vi "CHD-simulate-dashboard.vi"() -> ()   [LabVIEW 2019]
uses:
  Differential_Drive_System/CHD_DRIVE_GLOBALS.vi
  Simulation/CHS_SIM_SIM_Globals.vi
  Trajectory Following/CHS_TRAJECTORY_GLOBALS.vi
  Vision_Interface/CHS_Vision_Globals.vi
  <vilib>/Rock Robotics/WPI/ThirdParty/ChoreoLib/ChoreoLib.lvlib
  <vilib>/Rock Robotics/WPI/ThirdParty/JAS_Junk/TrajLib/TypeDef/ROTATION2D.ctl
  <vilib>/Rock Robotics/WPI/ThirdParty/JAS_Junk/TrajLib/Trajectory_Library.lvlib
  <vilib>/Rock Robotics/WPI/ThirdParty/JAS_Junk/TrajLib/TypeDef/CHASSIS_SPEEDS.ctl
  <vilib>/Rock Robotics/WPI/ThirdParty/JAS_Junk/TrajLib/TypeDef/TRANSLATION2D.ctl
  <vilib>/Rock Robotics/WPI/ThirdParty/JAS_Junk/TrajLib/TypeDef/POSE2D.ctl
panel:
  in  "Tab Control":T1(tab)
  out "Battery Voltage":dbl(graph)
  out "Swerve Motor Demands":T2(graph)
  out "Drive Motor Demands":T2(graph)
  out "Swerve Module Devices":T3(array[cluster])
  out "GyroReading_Degreees":dbl format="%15.3f"
  out "Encoder Distances":dbl[](array[numeric]) format="%17.2f"
  out "Encoder Velocities":dbl[](array[numeric]) format="%17.2f"
  out "Motor Demands":dbl[](array[numeric]) format="%17.2f"
  out "Battery Volts":dbl format="%16.2f"
  out "Mod Wheel \nSpeed Dmd":dbl[](array[numeric]) format="%17.3f"
  out "Swerve Drive Motor output":T4(graph)
  out "Drive Wheel Speed M/S":T5(graph)
  out "Swerve Drive Speed Error  M/S":T6(graph)
  out "Closed Loop Control":bool
  out "Orientation Angle Dmd_Rad":dbl format="%17.3f"
  out "Drv Chassis Adj Velocity DmD":T7 {"vOmega" format="%10.3f"; "vY" format="%10.3f"; "vX" format="%10.3f"}
  out "GyroHeading_Radians":dbl format="%17.2f"
  out "Orientation Angle Error_Rad":dbl format="%17.3f"
  out "Orientation Correct CO":dbl format="%17.3f"
  out "Swerve Chassis Speed":T7 {"vOmega" format="%10.3f"; "vY" format="%10.3f"; "vX" format="%10.3f"}
  out "Mod Wheel Out":dbl[](array[numeric]) format="%17.3f"
  out "Drive Wheel Speed M/S":dbl[](array[numeric]) format="%17.3f"
  out "Mod Wheel Speed Err":dbl[](array[numeric]) format="%17.3f"
  out "Mod Wheel \nSpeed Dmd":dbl[](array[numeric]) format="%17.3f"
  out "Closed Loop Control 2":bool
  out "Vision Pose":T8={"TRANSLATION"={"X"=0.0, "Y"=0.0}, "ROTATION"={"VALUE"=0.0, "COS"=1.0, "SIN"=0.0}} {"ROTATION"."SIN" format="%13.4f"; "ROTATION"."COS" format="%13.4f"; "ROTATION"."VALUE" format="%13.4f"; "TRANSLATION"."Y" format="%14.3f"; "TRANSLATION"."X" format="%14.3f"}
  out "Vision\nPose":bool
  out "Trajectory Status":T11(graph)
  out "Trajectory Execution \nClosed Loop":bool
  out "Trajectory Error":T12(graph)
  out "Traj_OnTarget":bool
  out "Traj Heading Dmd Deg":dbl format="%17.2f"
  out "Traj Final Heading Dmd Deg":dbl format="%17.2f"
  out "Traj Sample Time Sec":dbl format="%17.2f"
  out "Traj Rot Vel FF Rad/Sec":dbl format="%17.2f"
  out "Relative Trajectory Pose":T8={"TRANSLATION"={"X"=0.0, "Y"=0.0}, "ROTATION"={"VALUE"=0.0, "COS"=1.0, "SIN"=0.0}} {"ROTATION"."SIN" format="%13.4f"; "ROTATION"."COS" format="%13.4f"; "ROTATION"."VALUE" format="%13.4f"; "TRANSLATION"."Y" format="%14.3f"; "TRANSLATION"."X" format="%14.3f"}
  out "Absolute Odometry \nPose":T8={"TRANSLATION"={"X"=0.0, "Y"=0.0}, "ROTATION"={"VALUE"=0.0, "COS"=1.0, "SIN"=0.0}} {"ROTATION"."SIN" format="%13.4f"; "ROTATION"."COS" format="%13.4f"; "ROTATION"."VALUE" format="%13.4f"; "TRANSLATION"."Y" format="%14.3f"; "TRANSLATION"."X" format="%14.3f"}
  out "Other ABS Odometry\nPose":T8={"TRANSLATION"={"X"=0.0, "Y"=0.0}, "ROTATION"={"VALUE"=0.0, "COS"=1.0, "SIN"=0.0}} {"ROTATION"."SIN" format="%13.4f"; "ROTATION"."COS" format="%13.4f"; "ROTATION"."VALUE" format="%13.4f"; "TRANSLATION"."Y" format="%14.3f"; "TRANSLATION"."X" format="%14.3f"}
  out "Absolue Trajectory":cluster{dbl[], dbl[]}(graph)
  out "Other Trajectory":cluster{dbl[], dbl[]}(graph)
  out "error out":errorcluster
  # "SIMULATION"
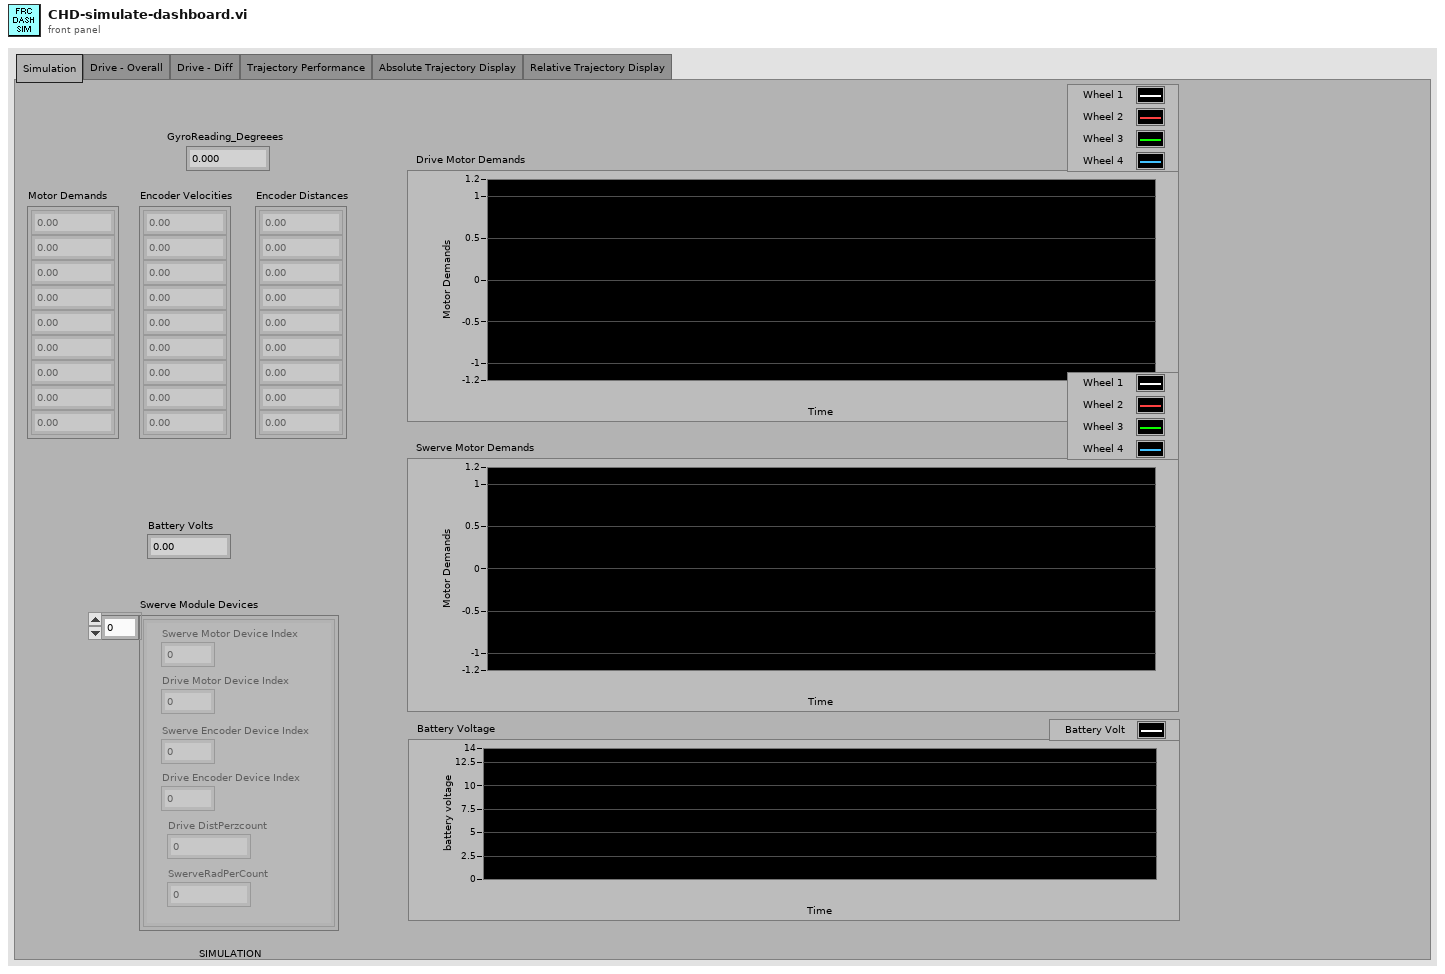
[diagram p1: front panel]
types:
  T1 = enum32{"Simulation", "Drive - Overall", "Drive - Diff", "Trajectory Performance", "Absolute Trajectory Display", "Relative Trajectory Display"}
  T2 = cluster{"Motor Dmd":dbl, "Motor Dmd":dbl, "Motor Dmd":dbl, "Motor Dmd":dbl}
  T3 = cluster{"Swerve Motor Device Index":i32, "Drive Motor Device Index":i32, "Swerve Encoder Device Index":i32, "Drive Encoder Device Index":i32, "Drive DistPerzcount":dbl, "SwerveRadPerCount":dbl}[]
  T4 = cluster{"Mod Wheel Out[0]":dbl, "Mod Wheel Out[1]":dbl, "Mod Wheel Out[2]":dbl, "Mod Wheel Out[3]":dbl}
  T5 = cluster{"LeftSpeed_MperS":dbl, "RightSpeed_MpserS":dbl}
  T6 = cluster{"Mod Wheel Speed Err[0]":dbl, "Mod Wheel Speed Err[1]":dbl, "Mod Wheel Speed Err[2]":dbl, "Mod Wheel Speed Err[3]":dbl}
  T7 = typedef "Trajectory_Library.lvlib/CHASSIS_SPEEDS.ctl" = cluster{"vX":dbl, "vY":dbl, "vOmega":dbl}
  T8 = typedef "Trajectory_Library.lvlib/POSE2D.ctl" = cluster{"TRANSLATION":T9, "ROTATION":T10}
  T9 = typedef "Trajectory_Library.lvlib/TRANSLATION2D.ctl" = cluster{"X":dbl, "Y":dbl}
  T10 = typedef "Trajectory_Library.lvlib/ROTATION2D.ctl" = cluster{"VALUE":dbl, "COS":dbl, "SIN":dbl}
  T11 = cluster{dbl, dbl, dbl, "Traj_Sample_Time_Sec":dbl}
  T12 = cluster{"Traj X Err":dbl, "Traj Y Err":dbl, "Traj Heading Err":dbl}
  T13 = cluster{"Traj X Err_FT":dbl, "Traj Y Err_FT":dbl, "Traj Heading Err_DEG":dbl}
  T14 = typedef "ChoreoLib.lvlib/ChoreoTrajectorySwerve.ctl" = cluster{"name":string, "samples":T15[], "splits":i32[], "events":T16[]}
  T15 = typedef "ChoreoLib.lvlib/ChoreoSwerveSample.ctl" = cluster{"timestamp":dbl, "x":dbl, "y":dbl, "heading":dbl, "velocityX":dbl, "velocityY":dbl, "angularVelocity":dbl, "accelX":dbl, "accelY":dbl, "accelAngular":dbl, "forceX":dbl[], "forceY":dbl[]}
  T16 = typedef "ChoreoLib.lvlib/ChoreoEventMarker.ctl" = cluster{"TimeStamp":dbl, "Name":string}
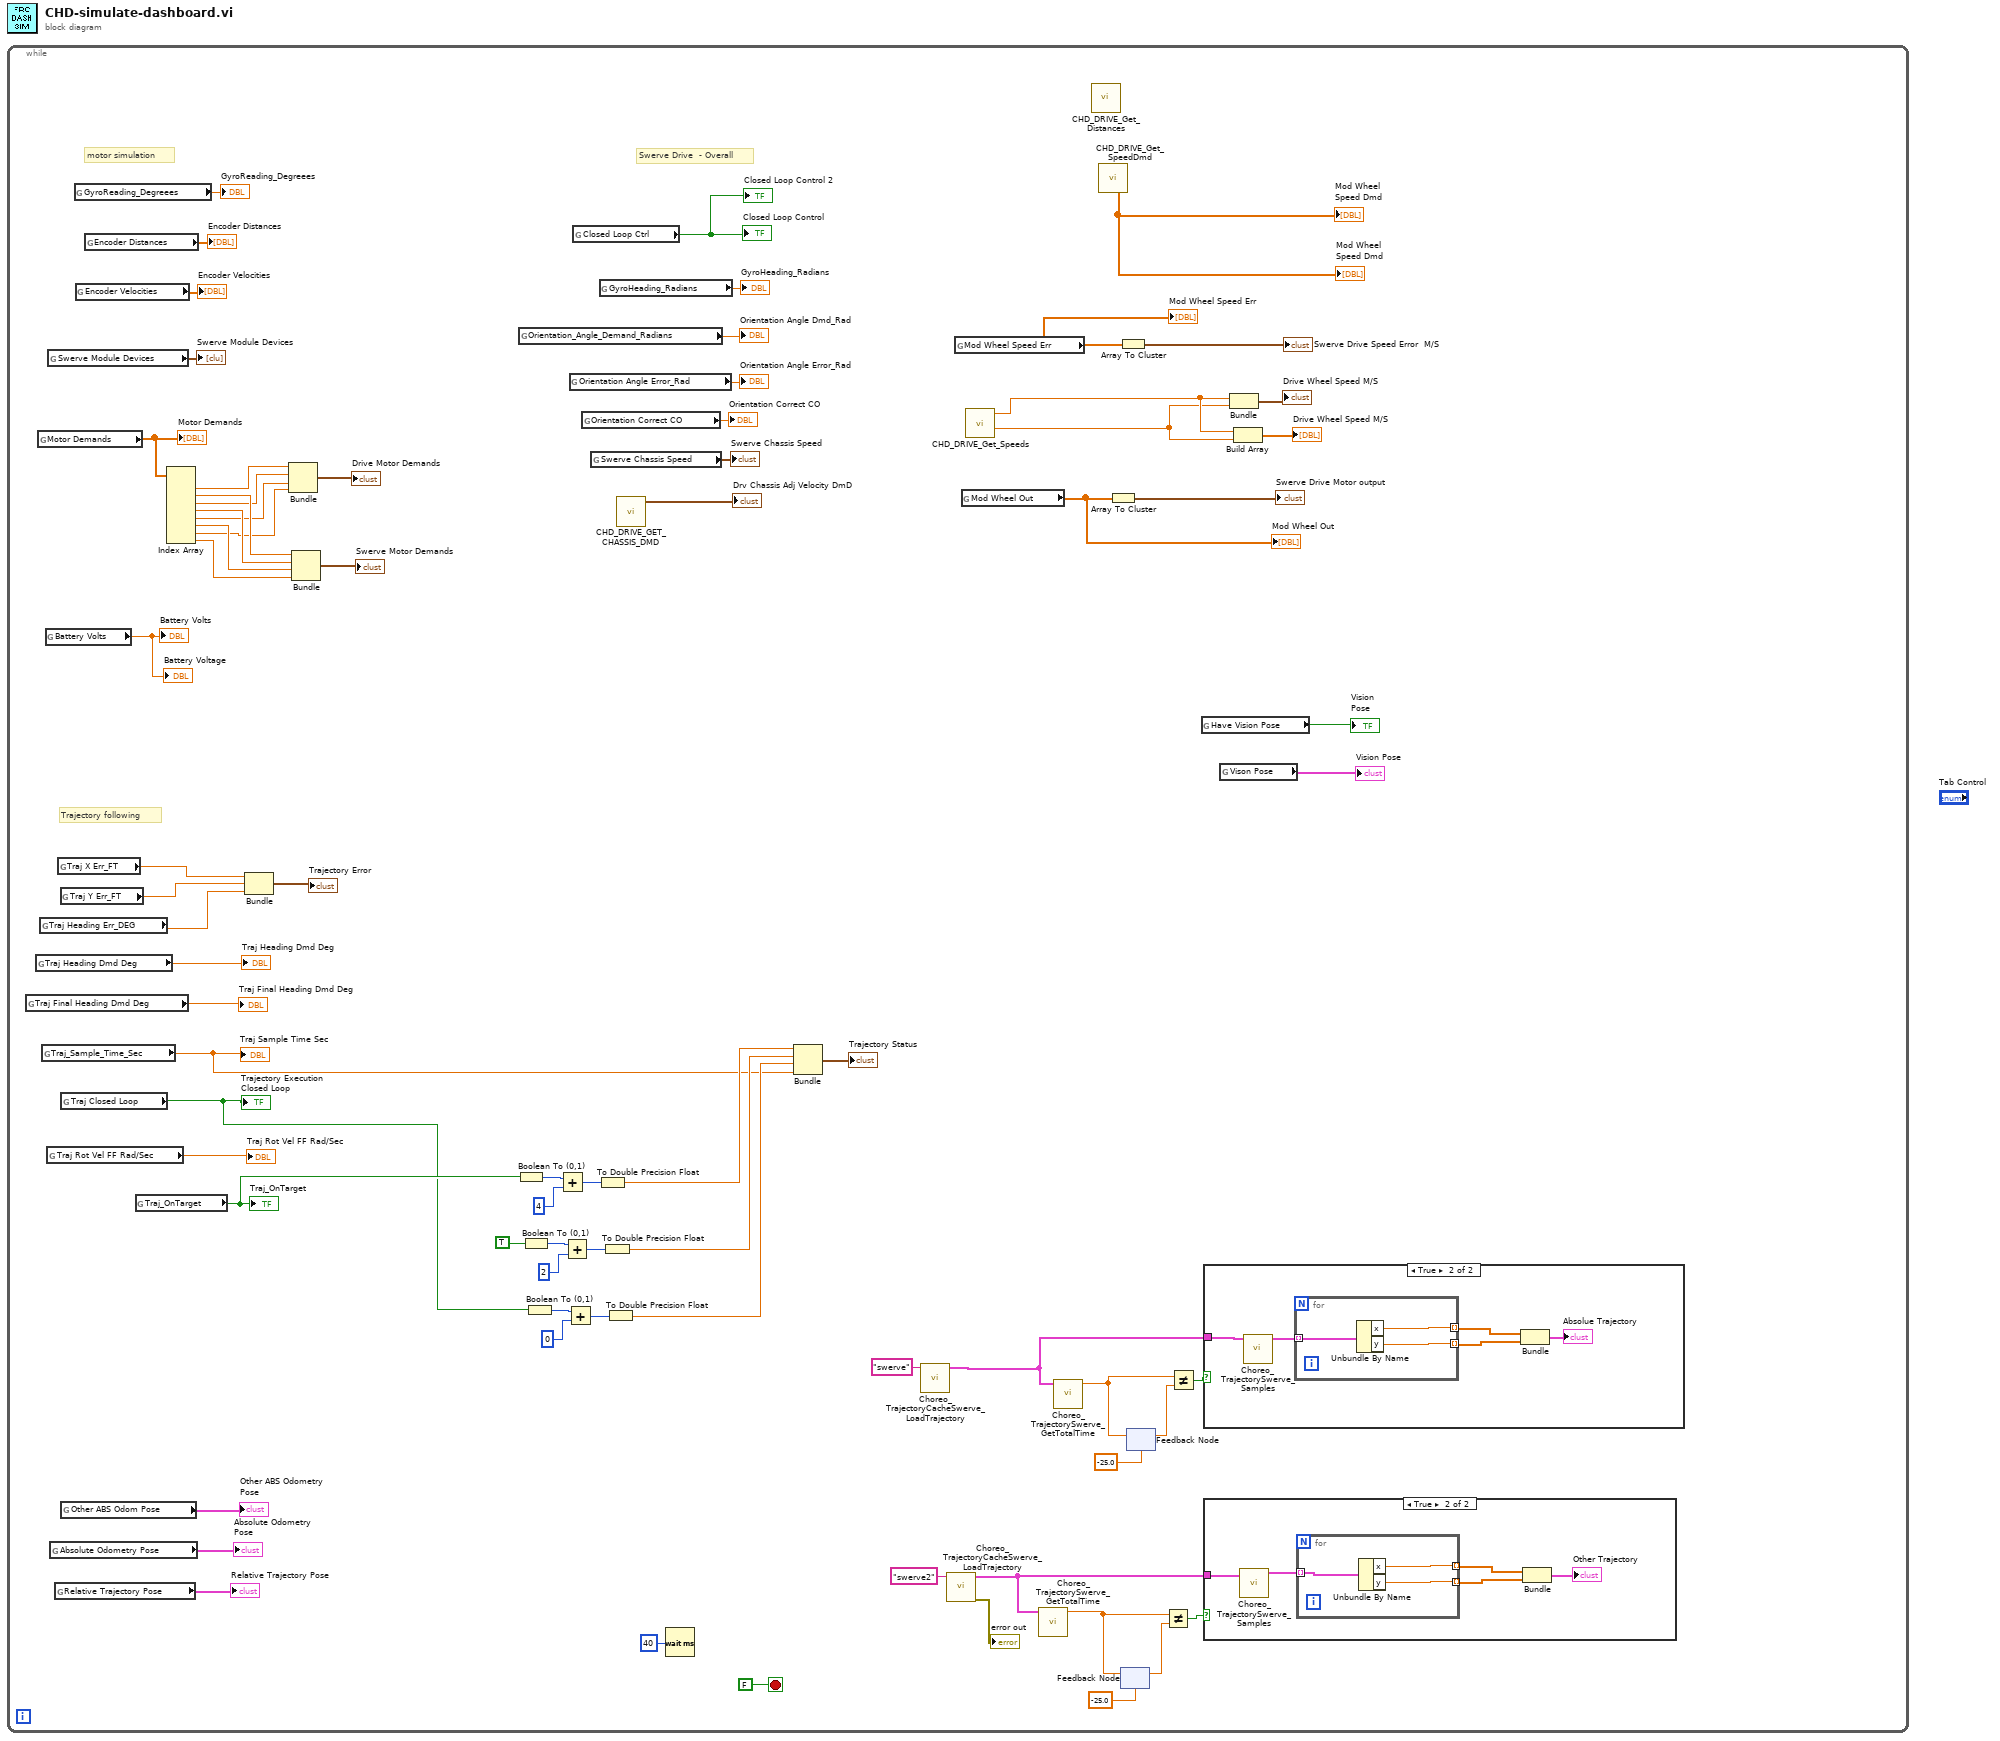
[diagram p0: block diagram]
diagram:
  n1 = while {
    stop <- FALSE stop-if-true
    # "Trajectory following"
    # "motor simulation"
    # "Swerve Drive  - Overall"
    n2 = global read "CHS_TRAJECTORY_GLOBALS.vi" "Traj Final Heading Dmd Deg"() -> (→"Traj Final Heading Dmd Deg":dbl)
    n3 = global read "CHS_TRAJECTORY_GLOBALS.vi" "Traj Heading Dmd Deg"() -> (→"Traj Heading Dmd Deg":dbl)
    n4 = global read "CHS_SIM_SIM_Globals.vi" "Motor Demands"() -> (w63:dbl[])
    "Motor Demands" <- w63
    n5 = global read "CHS_TRAJECTORY_GLOBALS.vi" "Traj Heading Err_DEG"() -> (w50:dbl)
    n6 = global read "CHS_TRAJECTORY_GLOBALS.vi" "Traj_Sample_Time_Sec"() -> (w31:dbl)
    "Traj Sample Time Sec" <- w31
    n7 = global read "CHS_SIM_SIM_Globals.vi" "Battery Volts"() -> (→"Battery Volts" →"Battery Voltage":dbl)
    n8 = global read "CHS_TRAJECTORY_GLOBALS.vi" "Traj Rot Vel FF Rad/Sec"() -> (→"Traj Rot Vel FF Rad/Sec":dbl)
    n9 = global read "CHS_SIM_SIM_Globals.vi" "Swerve Module Devices"() -> (→"Swerve Module Devices":T3)
    n10 = global read "CHS_TRAJECTORY_GLOBALS.vi" "Absolute Odometry Pose"() -> (→"Absolute Odometry \nPose":T8)
    n11 = global read "CHS_TRAJECTORY_GLOBALS.vi" "Relative Trajectory Pose"() -> (→"Relative Trajectory Pose":T8)
    n12 = global read "CHS_TRAJECTORY_GLOBALS.vi" "Traj X Err_FT"() -> (w52:dbl)
    n13 = global read "CHS_TRAJECTORY_GLOBALS.vi" "Traj Y Err_FT"() -> (w51:dbl)
    n14 = global read "CHS_TRAJECTORY_GLOBALS.vi" "Traj Closed Loop"() -> (w33:bool)
    "Trajectory Execution \nClosed Loop" <- w33
    n15 = global read "CHS_TRAJECTORY_GLOBALS.vi" "Other ABS Odom Pose"() -> (→"Other ABS Odometry\nPose":T8)
    n16 = global read "CHS_SIM_SIM_Globals.vi" "GyroReading_Degreees"() -> (→"GyroReading_Degreees":dbl)
    n17 = global read "CHS_SIM_SIM_Globals.vi" "Encoder Velocities"() -> (→"Encoder Velocities":dbl[])
    n18 = global read "CHS_SIM_SIM_Globals.vi" "Encoder Distances"() -> (→"Encoder Distances":dbl[])
    n19 = global read "CHS_TRAJECTORY_GLOBALS.vi" "Traj_OnTarget"() -> (w45:bool)
    "Traj_OnTarget" <- w45
    n20 = Index Array(array=w63) -> (element #1=w62:dbl, element #2=w61:dbl, element #3=w60:dbl, element #4=w59:dbl, element #5=w58:dbl, element #6=w57:dbl, element #7=w56:dbl, element #8=w55:dbl)  [unwired: 8 in]
    n21 = Bundle("Traj X Err_FT"=w52, "Traj Y Err_FT"=w51, "Traj Heading Err_DEG"=w50) -> (→"Trajectory Error":T13)  [unwired: 1 in]
    n22 = Bundle("Motor Dmd"=w62, "Motor Dmd"=w60, "Motor Dmd"=w58, "Motor Dmd"=w56) -> (→"Drive Motor Demands":T2)  [unwired: 1 in]
    n23 = Bundle("Motor Dmd"=w61, "Motor Dmd"=w59, "Motor Dmd"=w57, "Motor Dmd"=w55) -> (→"Swerve Motor Demands":T2)  [unwired: 1 in]
    n24 = Boolean To (0,1)(Boolean=w45) -> (0, 1=w43:i16)
    n25 = global read "CHD_DRIVE_GLOBALS.vi" "Orientation_Angle_Demand_Radians"() -> (→"Orientation Angle Dmd_Rad":dbl)
    n26 = Boolean To (0,1)(Boolean=TRUE) -> (0, 1=w40:i16)
    n27 = Boolean To (0,1)(Boolean=w33) -> (0, 1=w36:i16)
    n28 = Add(x=w43, y=i16 4) -> (x+y=w42:i16)
    n29 = Add(x=w40, y=i16 2) -> (x+y=w39:i16)
    n30 = Add(x=w36, y=i16 0) -> (x+y=w35:i16)
    n31 = global read "CHD_DRIVE_GLOBALS.vi" "Orientation Angle Error_Rad"() -> (→"Orientation Angle Error_Rad":dbl)
    n32 = global read "CHD_DRIVE_GLOBALS.vi" "Closed Loop Ctrl"() -> (→"Closed Loop Control" →"Closed Loop Control 2":bool)
    n33 = global read "CHD_DRIVE_GLOBALS.vi" "Orientation Correct CO"() -> (→"Orientation Correct CO":dbl)
    n34 = global read "CHD_DRIVE_GLOBALS.vi" "Swerve Chassis Speed"() -> (→"Swerve Chassis Speed":T7)
    n35 = To Double Precision Float(number=w42) -> (double precision float=w44:dbl)
    n36 = global read "CHD_DRIVE_GLOBALS.vi" "GyroHeading_Radians"() -> (→"GyroHeading_Radians":dbl)
    n37 = To Double Precision Float(number=w39) -> (double precision float=w37:dbl)
    n38 = To Double Precision Float(number=w35) -> (double precision float=w32:dbl)
    n39 = call "CHD_DRIVE_GET_CHASSIS_DMD.vi"() -> ("Drv Chassis Velocity DmD"=→"Drv Chassis Adj Velocity DmD":T7)  [unwired: 11 in]
    n40 = Wait (ms)(milliseconds to wait=u32 40) -> ()  [unwired: 1 out]
    n41 = Bundle(w44, w37, w32, "Traj_Sample_Time_Sec"=w31) -> (→"Trajectory Status":T11)  [unwired: 1 in]
    n42 = call <vilib>:"Choreo_TrajectoryCacheSwerve_LoadTrajectory.vi"("TrajectoryName"="swerve") -> ("ChoreoTrajectorySwerve"=w10:T14)  [unwired: 9 in, 1 out]
    n43 = call <vilib>:"Choreo_TrajectoryCacheSwerve_LoadTrajectory.vi"("TrajectoryName"="swerve2") -> ("error out"=→"error out":errorcluster, "ChoreoTrajectorySwerve"=w7:T14)  [unwired: 9 in]
    n44 = global read "CHD_DRIVE_GLOBALS.vi" "Mod Wheel Speed Err"() -> (w26:dbl[])
    "Mod Wheel Speed Err" <- w26
    n45 = global read "CHD_DRIVE_GLOBALS.vi" "Mod Wheel Out"() -> (w23:dbl[])
    "Mod Wheel Out" <- w23
    n46 = call "CHD_DRIVE_Get_Speeds.vi"() -> ("RightSpeed_MpserS"=w3:dbl, "LeftSpeed_MperS"=w4:dbl)  [unwired: 9 in, 1 out]
    n47 = call <vilib>:"Choreo_TrajectorySwerve_GetTotalTime.vi"("ChoreoTrajectorySwerve"=w7) -> ("TotalTime"=w11:dbl)  [unwired: 10 in]
    n48 = call <vilib>:"Choreo_TrajectorySwerve_GetTotalTime.vi"("ChoreoTrajectorySwerve"=w10) -> ("TotalTime"=w12:dbl)  [unwired: 10 in]
    n49 = call "CHD_DRIVE_Get_Distances.vi"() -> ()  [unwired: 9 in, 3 out]
    n50 = call "CHD_DRIVE_Get_SpeedDmd.vi"() -> ("MotorSpeedDmds_MperSec"=→"Mod Wheel \nSpeed Dmd" →"Mod Wheel \nSpeed Dmd":dbl[])  [unwired: 9 in, 2 out]
    n51 = Array To Cluster(array=w23) -> (cluster=→"Swerve Drive Motor output":T4)
    n52 = Array To Cluster(array=w26) -> (cluster=→"Swerve Drive Speed Error  M/S":T6)
    n53 = feedback #1(-25.0 ("TotalTime_Sec")) -> (w14:dbl)
    n54 = feedback-in #1(w11) -> ()
    n55 = feedback #2(-25.0 ("TotalTime_Sec")) -> (w17:dbl)
    n56 = feedback-in #2(w12) -> ()
    n57 = Not Equal?(x=w11, y=w14) -> (x != y?=w13:bool)
    n58 = Not Equal?(x=w12, y=w17) -> (x != y?=w16:bool)
    n59 = global read "CHS_Vision_Globals.vi" "Have Vision Pose"() -> (→"Vision\nPose":bool)
    n60 = case shown="True" w13 {
      tunnel: w7 -> [_ w78]
      frame False {
      }
      frame True {
        n61 = call <vilib>:"Choreo_TrajectorySwerve_Samples.vi"("ChoreoTrajectorySwerve"=w78) -> ("samples"=w77:T15[])  [unwired: 10 in]
        n62 = for {
          tunnel: [w84] -> w80 mode=indexing
          tunnel: [w83] -> w81 mode=indexing
          tunnel: w77 -> [w82] mode=indexing
          n63 = Unbundle By Name(w82) -> ("x"=w84:dbl, "y"=w83:dbl)
        }
        n64 = Bundle(w80, w81) -> (→"Other Trajectory":cluster{dbl[], dbl[]})  [unwired: 1 in]
      }
    }
    n65 = case shown="True" w16 {
      tunnel: w10 -> [_ w86]
      frame False {
      }
      frame True {
        n66 = call <vilib>:"Choreo_TrajectorySwerve_Samples.vi"("ChoreoTrajectorySwerve"=w86) -> ("samples"=w85:T15[])  [unwired: 10 in]
        n67 = for {
          tunnel: [w92] -> w88 mode=indexing
          tunnel: [w91] -> w89 mode=indexing
          tunnel: w85 -> [w90] mode=indexing
          n68 = Unbundle By Name(w90) -> ("x"=w92:dbl, "y"=w91:dbl)
        }
        n69 = Bundle(w88, w89) -> (→"Absolue Trajectory":cluster{dbl[], dbl[]})  [unwired: 1 in]
      }
    }
    n70 = global read "CHS_Vision_Globals.vi" "Vison Pose"() -> (→"Vision Pose":T8)
    n71 = Bundle("LeftSpeed_MperS"=w4, "RightSpeed_MpserS"=w3) -> (→"Drive Wheel Speed M/S":T5)  [unwired: 1 in]
    n72 = Build Array(w4, w3) -> (→"Drive Wheel Speed M/S":dbl[])
  }
